vi "createCommandList.vi"(8 "error in (no error)":errorcluster, 10 "Parameters":u32[](array[numeric]), 11 "Burst in":refnum<class "Burst.lvclass">) -> (0 "error out":errorcluster, 2 "Commandlist":string, 3 "Burst out":refnum<class "Burst.lvclass">)   [LabVIEW 2013, in "Burst.lvclass"]
uses:
  Burst.lvclass
  lib/Utilities.lvlib
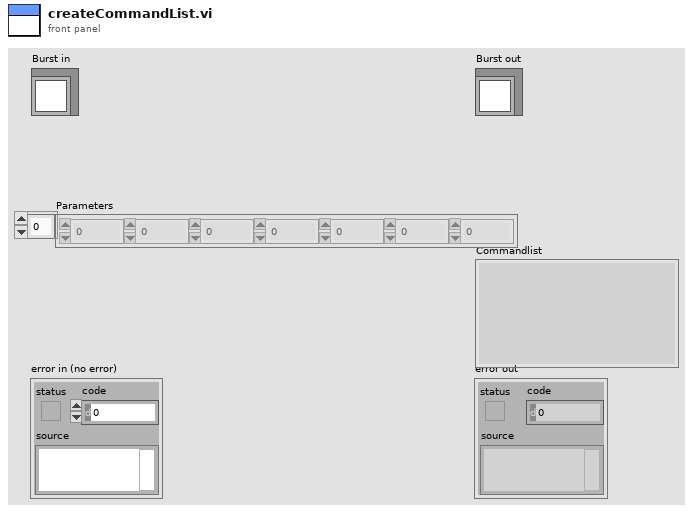
[diagram p1: front panel]
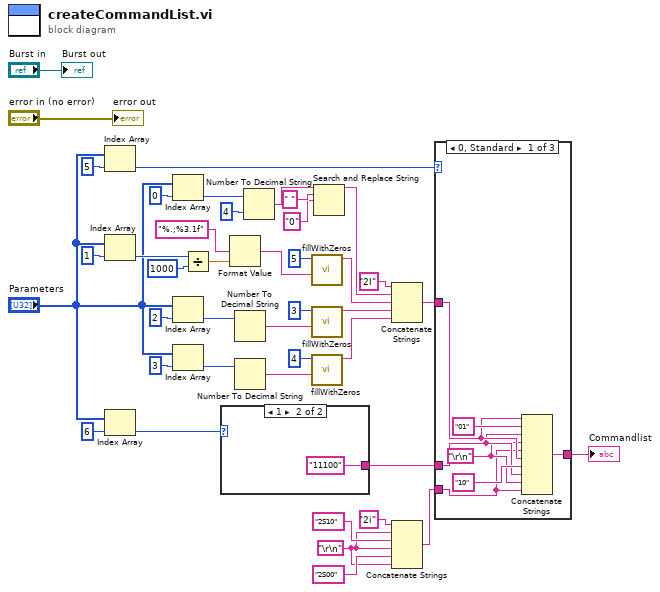
[diagram p0: block diagram]
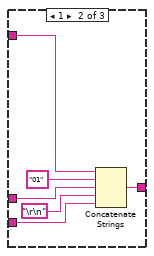
[diagram p2: hidden frame]
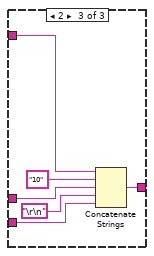
[diagram p3: hidden frame]
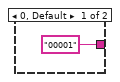
[diagram p4: hidden frame]
diagram:
  w2 = "\r\n"
  n1 = Index Array(array="Parameters", index=5) -> (element=w9:u32)
  n2 = Index Array(array="Parameters", index=1) -> (element=w30:u32)
  n3 = Index Array(array="Parameters", index=6) -> (element=w10:u32)
  n4 = Index Array(array="Parameters", index=0) -> (element=w38:u32)
  n5 = Index Array(array="Parameters", index=2) -> (element=w22:u32)
  n6 = Index Array(array="Parameters", index=3) -> (element=w16:u32)
  n7 = Divide(x=w30, y=u32 1000) -> (x/y=w28:dbl)
  n8 = case shown="1" w10 {
    tunnel: ["00001" "11100"] -> w7
    frame 0, Default {
    }
    frame 1 {
    }
  }
  n9 = Format Value(format string="%.;%3.1f", value (0)=w28) -> (output string=w25:string)  [unwired: 1 in]
  n10 = Number To Decimal String(number=w22) -> (decimal integer string=w21:string)  [unwired: 1 in]
  n11 = Number To Decimal String(number=w16) -> (decimal integer string=w17:string)  [unwired: 1 in]
  n12 = Number To Decimal String(number=w38, width (-)=i16 4) -> (decimal integer string=w36:string)
  n13 = call "fillWithZeros.vi"("string in"=w25, "width"=5 ("x")) -> ("string out"=w24:string)  [unwired: 9 in]
  n14 = call "fillWithZeros.vi"("string in"=w21, "width"=3) -> ("string out"=w19:string)  [unwired: 9 in]
  n15 = call "fillWithZeros.vi"("string in"=w17, "width"=4) -> ("string out"=w14:string)  [unwired: 9 in]
  n16 = Search and Replace String(input string=w36, search string=" ", replace string="0" ("replace string (\"\")")) -> (result string=w33:string)  [unwired: 5 in, 3 out]
  n17 = Concatenate Strings("2I", w33, w24, w19, w14) -> (w8:string)
  n18 = Concatenate Strings("2i" ("String"), w2, "2S10", w2, "2S00", w2) -> (w1:string)
  n19 = case shown="0, Standard" w9 {
    tunnel: w8 -> [w48 w56 w62]
    tunnel: w7 -> [w46 w54 w61]
    tunnel: [w49 w53 w59] -> w6
    tunnel: w1 -> [w44 w51 w57]
    frame 0, Default {
      w45 = "\r\n"
      n20 = Concatenate Strings(w48, "01" ("string"), w46, w45, w44, w48, "10" ("string"), w46, w45, w44) -> (w49:string)
    }
    frame 1 {
      n21 = Concatenate Strings(w56, "01" ("string"), w54, "\r\n", w51) -> (w53:string)
    }
    frame 2 {
      n22 = Concatenate Strings(w62, "10" ("string"), w61, "\r\n", w57) -> (w59:string)
    }
  }
  "Commandlist" <- w6
  "error out" <- "error in (no error)"
  "Burst out" <- "Burst in"
